vi "sql_q.vi"(4 "error in":errorcluster, 6 "SQL query":string, 7 "connect ref":T1) -> (0 "error out":errorcluster, 1 "recordset data":variant[][](array[variant]), 2 "Columns":string[](array[string]), 3 "conn ref out":T1)   [LabVIEW 2010]
uses:
  <vilib>/addons/database/Connection.llb/Conn ObjectReference.ctl
  <vilib>/addons/database/Connection.llb/Conn Execute.vi
  <vilib>/addons/database/Recordset.llb/Rec Get Recordset Properties (R).vi
  <vilib>/addons/database/Recordset.llb/Rec Fetch Recordset Data (R).vi
  <vilib>/addons/database/Recordset.llb/Rec Destroy - Connection.vi
  <vilib>/addons/database/Recordset.llb/Rec Get Column Properties (R).vi
  <vilib>/addons/database/NI_Database_API.lvlib
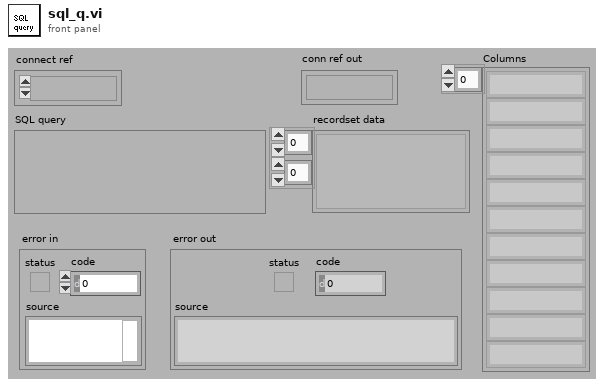
[diagram p1: front panel]
types:
  T1 = typedef "NI_Database_API.lvlib/Conn ObjectReference.ctl" = refnum<k1>
  T2 = typedef "NI_Database_API.lvlib/Rec ObjectReference.ctl" = refnum<k1>
  T3 = typedef "NI_Database_API.lvlib/Rec Properties.ctl" = cluster{"column count":i32, "record index":i32, "record count":i32, "bof?":bool, "eof?":bool, "cursor type":T4, "cache size":i32, "state":enum16{"closed", "open"}}
  T4 = typedef "NI_Database_API.lvlib/DB Tools Cursor Type.ctl" = enum16{"forward-only", "keyset", "dynamic", "static"}
  T5 = typedef "NI_Database_API.lvlib/Rec Column Properties.ctl" = cluster{"name":string, "database data type":T6, "defined size":i32, "actual size":i32}
  T6 = typedef "NI_Database_API.lvlib/DB Tools DataTypes.ctl" = enum16{"String", "Long (I32)", "Single (SGL)", "Double (DBL)", "Date/Time", "Binary"}
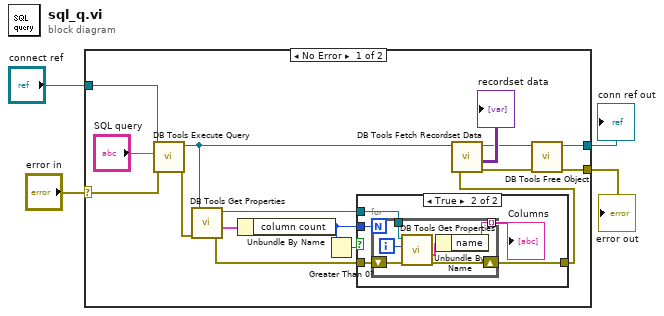
[diagram p0: block diagram]
diagram:
  n1 = case shown="No Error" "error in" {
    selector: "error in" -> [w5 w33]
    tunnel: "connect ref" -> [w20 w34]
    tunnel: [w18 w34] -> w3
    tunnel: [w17 w33] -> w2
    frame No Error {
      n2 = call-poly <vilib>:"DB Tools Execute Query.vi"("error in (no error)"=w5, "SQL query"="SQL query", "connection reference"=w20) -> ("error out"=w7:errorcluster, "recordset reference"=w8:T2)  [unwired: 5 in]
      n3 = call-poly <vilib>:"DB Tools Get Properties.vi"("error in (no error)"=w7, "recordset reference"=w8) -> ("error out"=w14:errorcluster, "recordset properties"=w16:T3, "recordset reference out"=w15:T2)  [unwired: 3 in]
      n4 = Unbundle By Name(w16) -> ("column count"=w13:i32)
      n5 = Greater Than 0?(x=w13) -> (x > 0?=w9:bool)
      n6 = case shown="True" w9 {
        tunnel: w13 -> [_ w26]
        tunnel: w15 -> [_ w25]
        tunnel: w14 -> [w21 w24]
        tunnel: [w21 w22] -> w6
        frame False {
        }
        frame True {
          n7 = for {
            N: w26 -> [_]
            tunnel: w25 -> [w32]
            tunnel: [w28] -> w23 mode=indexing
            shift-right: [w27] -> w22
            shift-left: w24 -> [w31]
            i -> [w29]
            n8 = call-poly <vilib>:"DB Tools Get Properties.vi"("error in (no error)"=w31, "column index"=w29, "recordset reference"=w32) -> ("error out"=w27:errorcluster, "column properties"=w30:T5)  [unwired: 2 in, 1 out]
            n9 = Unbundle By Name(w30) -> ("name"=w28:string)
          }
          "Columns" <- w23
        }
      }
      n10 = call-poly <vilib>:"DB Tools Fetch Recordset Data.vi"("error in (no error)"=w6, "recordset reference"=w8) -> ("error out"=w10:errorcluster, "recordset data"=→"recordset data":variant[][], "recordset reference out"=w11:T2)  [unwired: 3 in]
      n11 = call-poly <vilib>:"DB Tools Free Object.vi"("error in (no error)"=w10, "recordset reference"=w11) -> ("error out"=w17:errorcluster, "connection reference"=w18:T1)  [unwired: 8 in]
    }
    frame Error {
    }
  }
  "conn ref out" <- w3
  "error out" <- w2
